vi "AFXP Main.vi"() -> ()   [LabVIEW 2015]
doc: "Simple File Manager for the Adafruid Audio FX Sound Board\nhttps://learn.adafruit.com/adafruit-audio-fx-sound-board/overview"
uses:
  controls/AFXP State.ctl
  controls/AFXP Data.ctl
  controls/AFCP Setup.ctl
  <vilib>/Utility/error.llb/DialogType.ctl
  <userlib>/_OpenG.lib/file/file.llb/File Exists - Scalar__ogtk.vi
panel:
  in  "Clear Button":bool
  in  "Button Ctrl":T1={"Trigger Type:"=enum."Disabled", "Sound Files"=[]}
  in  "Folder Drop":path
  in  "Prev Button":bool
  in  "Next Button":bool
  in  "Button Selection":T2(ring)
  in  "Make Button":bool
  in  "Destination":path
  # "AUDIO FILE LIST"
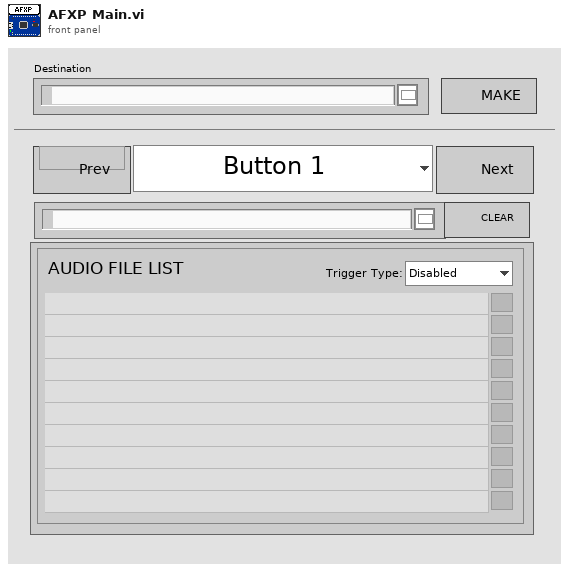
[diagram p1: front panel]
types:
  T1 = cluster{"Trigger Type:":enum16{"Basic", "Hold-Loop", "Latch-Loop", "Next", "Random", "Disabled"}, "Sound Files":path[]}
  T2 = enum8{"Button 1", "Button 2", "Button 3", "Button 4", "Button 5", "Button 6", "Button 7", "Button 8", "Button 9", "Button 10", "Button 11", "Button 12"}
  T3 = typedef "AFXP Data.ctl" = cluster{"changes_saved?":bool, "button_setup":T4[], "Destination":path}
  T4 = typedef "AFCP Setup.ctl" = cluster{"trigger":enum16{"Basic", "Hold-Loop", "Latch-Loop", "Next", "Random", "Disabled"}, "files":path[]}
  T5 = typedef "AFXP State.ctl" = enum16{"Initialize", "Wait for Event", "Make", "Load", "Save", "Folder Drop", "Prev", "Next", "Button Ctrl", "Destination", "Selection", "Exit"}
  T6 = cluster{"Trigger Type":enum16{"Basic", "Hold-Loop", "Latch-Loop", "Next", "Random", "Disabled"}, "Sound Files":path[]}
  T7 = typedef "DialogType.ctl" = u16
  T8 = cluster{"Trigger Type":enum16{"Basic", "Hold-Loop", "Latch-Loop", "Next", "Random", "Disabled"}, "Sound Files":path[]}[]
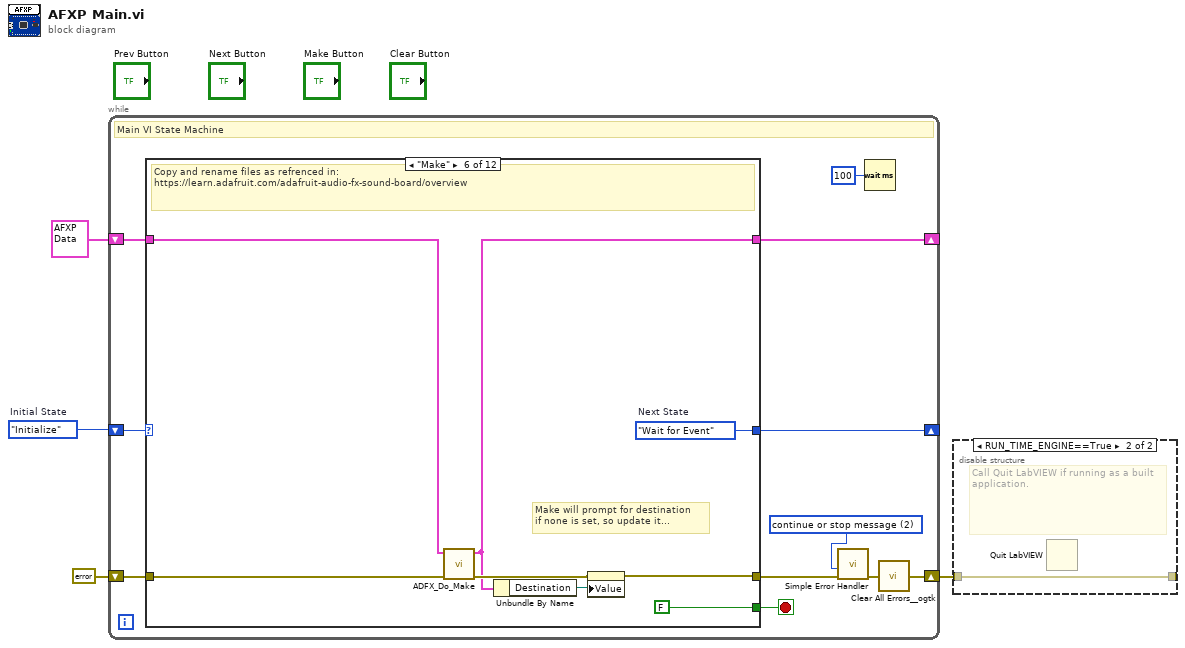
[diagram p0: block diagram]
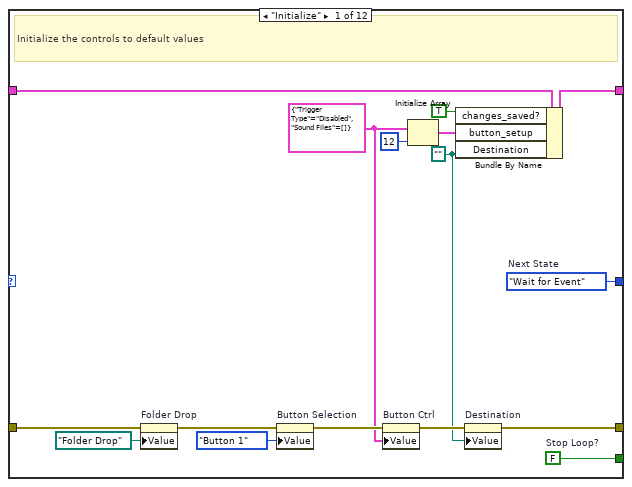
[diagram p2: hidden frame]
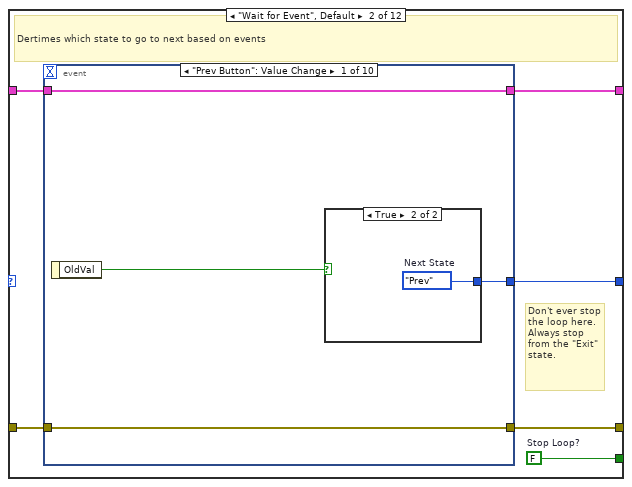
[diagram p3: hidden frame]
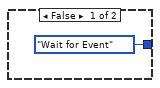
[diagram p4: hidden frame]
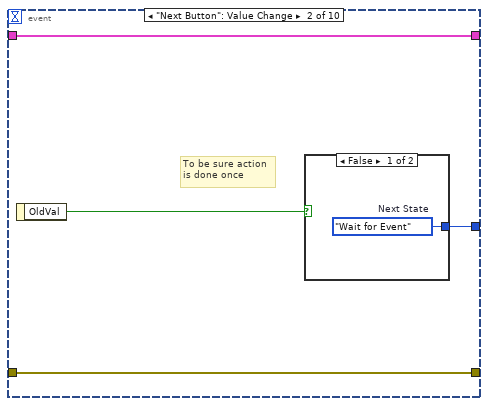
[diagram p5: hidden frame]
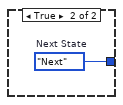
[diagram p6: hidden frame]
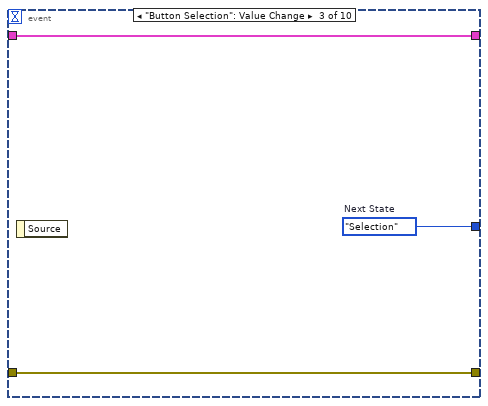
[diagram p7: hidden frame]
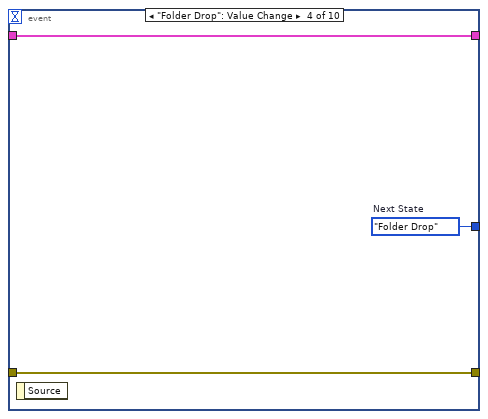
[diagram p8: hidden frame]
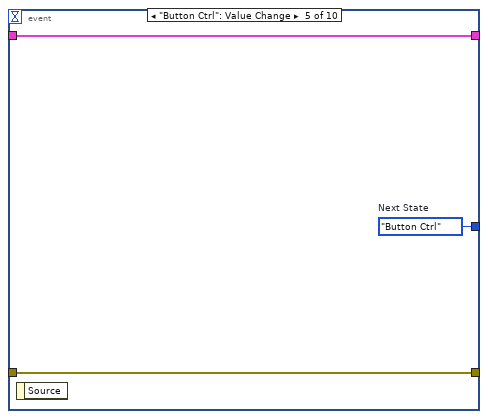
[diagram p9: hidden frame]
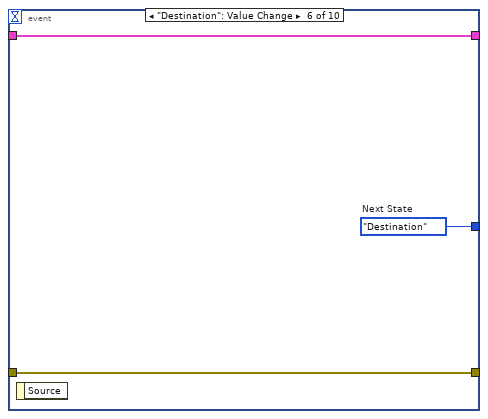
[diagram p10: hidden frame]
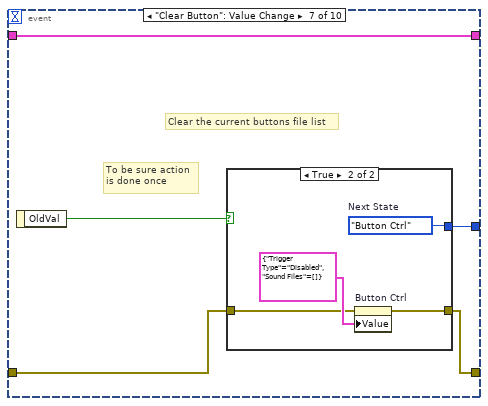
[diagram p11: hidden frame]
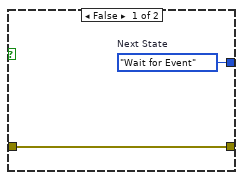
[diagram p12: hidden frame]
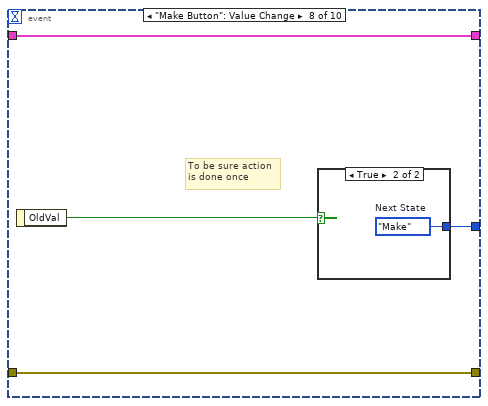
[diagram p13: hidden frame]
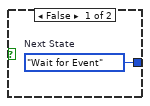
[diagram p14: hidden frame]
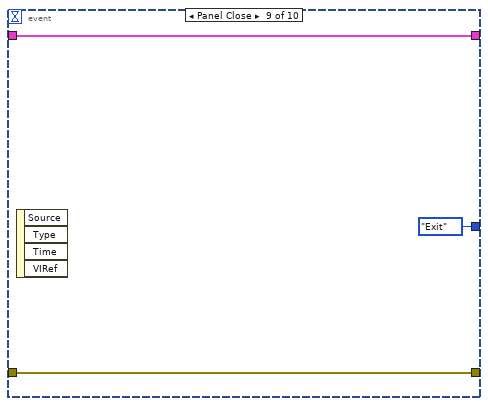
[diagram p15: hidden frame]
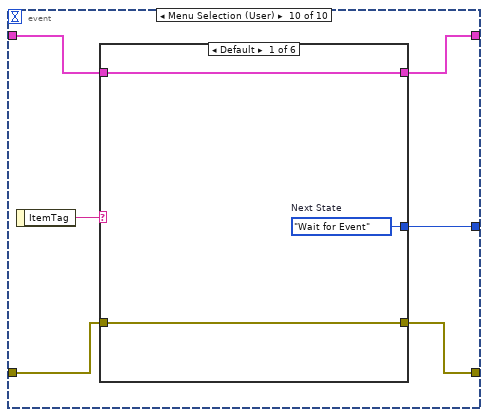
[diagram p16: hidden frame]
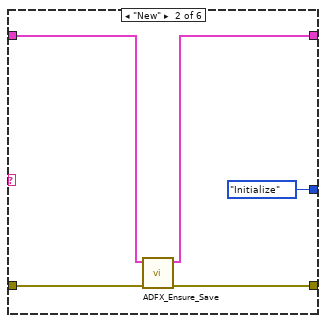
[diagram p17: hidden frame]
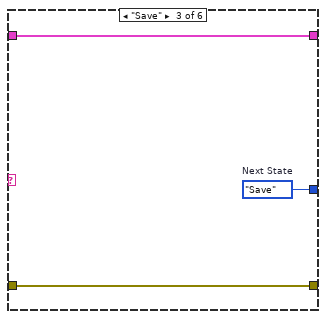
[diagram p18: hidden frame]
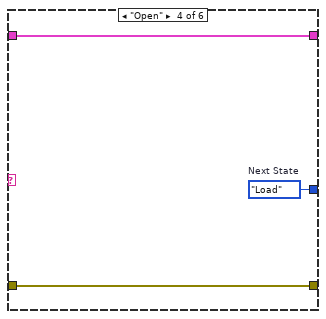
[diagram p19: hidden frame]
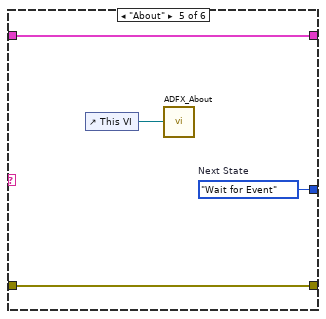
[diagram p20: hidden frame]
diagram:
  w4 = AFXP_State."Initialize"  # Initial State
  n1 = while {
    shift-right: [w14] -> _
    shift-left: w4 -> [w15]
    shift-right: [w12] -> _
    shift-left: T3 {"changes_saved?"=TRUE, "button_setup"=[{"trigger"=enum."Basic", "files"=[]}, {"trigger"=enum."Basic", "files"=[]}, {"trigger"=enum."Basic", "files"=[]}, {"trigger"=enum."Basic", "files"=[]}, {"trigger"=enum."Basic", "files"=[]}, {"trigger"=enum."Basic", "files"=[]}, {"trigger"=enum."Basic", "files"=[]}, {"trigger"=enum."Basic", "files"=[]}, {"trigger"=enum."Basic", "files"=[]}, {"trigger"=enum."Basic", "files"=[]}, {"trigger"=enum."Basic", "files"=[]}, {"trigger"=enum."Basic", "files"=[]}, {"trigger"=enum."Basic", "files"=[]}], "Destination"=path ""} ("Data") -> [w13]
    shift-right: [w5] -> w1
    shift-left: errorcluster {"status"=FALSE, "code"=0, "source"=""} ("error constant") -> [w11]
    stop <- w6 stop-if-true
    w7 = T7 2 items=["no dialog", "OK message", "continue or stop message", "OK message + warnings", "continue/stop + warnings"] ("type of dialog (OK msg:1)")
    # "Main VI State Machine"
    n2 = case shown="\"Make\"" w15 {
      tunnel: [w31 w37 w114 w115 w133 w142 w160 w170 w171 w179 w187 w206] -> w14
      tunnel: [w30 w36 FALSE ("Stop Loop?") FALSE ("Stop Loop?") FALSE ("Stop Loop?") FALSE ("Stop Loop?") FALSE ("Stop Loop?") w169 FALSE ("Stop Loop?") FALSE ("Stop Loop?") FALSE ("Stop Loop?") FALSE ("Stop Loop?")] -> w6
      tunnel: w13 -> [w24 w35 w110 w120 w134 w139 w158 w166 w178 w186 w198 w205]
      tunnel: [w23 w34 w109 w116 w132 w136 w158 w165 w178 w186 w197 w205] -> w12
      tunnel: w11 -> [w29 w33 w111 w122 w126 w140 w157 w168 w176 w182 w194 w202]
      tunnel: [w17 w32 w112 w118 w125 w137 w151 w167 w172 w180 w191 w204] -> w9
      frame "Initialize" {
        w16 = path ""
        w20 = T6 {"Trigger Type"=enum."Disabled", "Sound Files"=[]} ("Button Ctrl")
        w30 = FALSE  # Stop Loop?
        w31 = AFXP_State."Wait for Event"  # Next State
        # "Initialize the controls to default values"
        n3 = property on="Folder Drop" class="Path"(error in=w29, "Value"=path "Folder Drop" ("Destination")) -> (error out=w26:errorcluster)  [unwired: 1 in, 1 out]
        n4 = property on="Button Selection" class="Enum (strict)"(error in=w26, "Value"=T2."Button 1" ("Button Selection")) -> (error out=w25:errorcluster)  [unwired: 1 in, 1 out]
        n5 = property on="Button Ctrl" class="Clust (strict)"(error in=w25, "Value"=w20) -> (error out=w18:errorcluster)  [unwired: 1 in, 1 out]
        n6 = Initialize Array(w20, 12 ("dimension size")) -> (w21:T8)
        n7 = Bundle By Name(cluster=w24, "changes_saved?"=TRUE, "button_setup"=w21, "Destination"=w16) -> (w23:T3)
        n8 = property on="Destination" class="Path"(error in=w18, "Value"=w16) -> (error out=w17:errorcluster)  [unwired: 1 in, 1 out]
      }
      frame "Wait for Event", Default {
        w36 = FALSE  # Stop Loop?
        # "Don't ever stop the loop here. Always stop from the \"Exit\" state."
        # "Dertimes which state to go to next based on events"
        n9 = event shown="[0] \"Prev Button\": Value Change" {
          selector: _ -> [_ _ _ _ _ _ _ _ _ _]
          dyn-events: _ -> [_ _ _ _ _ _ _ _ _ _]
          timeout: _ -> [_ _ _ _ _ _ _ _ _ _]
          tunnel: [w41 w45 w50 w53 w56 w59 w65 w74 AFXP_State."Exit" ("Next State") w86] -> w37
          tunnel: w35 -> [w40 w47 w52 w55 w58 w61 w66 w76 w81 w83]
          tunnel: [w40 w47 w52 w55 w58 w61 w66 w76 w81 w82] -> w34
          tunnel: w33 -> [w39 w46 w51 w54 w57 w60 w63 w75 w80 w85]
          tunnel: [w39 w46 w51 w54 w57 w60 w62 w75 w80 w84] -> w32
          event "Prev Button": Value Change {
            n10 = event-data() -> ("OldVal"=w38:bool)  [unwired: 1 in]
            n11 = case shown="True" w38 {
              tunnel: [AFXP_State."Wait for Event" ("Next State") w43] -> w41
              frame False {
              }
              frame True {
                w43 = AFXP_State."Prev"  # Next State
              }
            }
          }
          event "Next Button": Value Change {
            # "To be sure action\nis done once"
            n12 = event-data() -> ("OldVal"=w44:bool)  [unwired: 1 in]
            n13 = case shown="False" w44 {
              tunnel: [w48 w49] -> w45
              frame False {
                w48 = AFXP_State."Wait for Event"  # Next State
              }
              frame True {
                w49 = AFXP_State."Next"  # Next State
              }
            }
          }
          event "Button Selection": Value Change {
            w50 = AFXP_State."Selection"  # Next State
            n14 = event-data() -> ()  [unwired: 1 in, 1 out]
          }
          event "Folder Drop": Value Change {
            w53 = AFXP_State."Folder Drop"  # Next State
            n15 = event-data() -> ()  [unwired: 1 in, 1 out]
          }
          event "Button Ctrl": Value Change {
            w56 = AFXP_State."Button Ctrl"  # Next State
            n16 = event-data() -> ()  [unwired: 1 in, 1 out]
          }
          event "Destination": Value Change {
            w59 = AFXP_State."Destination"  # Next State
            n17 = event-data() -> ()  [unwired: 1 in, 1 out]
          }
          event "Clear Button": Value Change {
            # "To be sure action\nis done once"
            # "Clear the current buttons file list"
            n18 = event-data() -> ("OldVal"=w64:bool)  [unwired: 1 in]
            n19 = case shown="True" w64 {
              tunnel: [w68 w72] -> w65
              tunnel: w63 -> [w67 w70]
              tunnel: [w67 w69] -> w62
              frame False {
                w68 = AFXP_State."Wait for Event"  # Next State
              }
              frame True {
                w72 = AFXP_State."Button Ctrl"  # Next State
                n20 = property on="Button Ctrl" class="Clust (strict)"(error in=w70, "Value"=T6 {"Trigger Type"=enum."Disabled", "Sound Files"=[]} ("Button Ctrl")) -> (error out=w69:errorcluster)  [unwired: 1 in, 1 out]
              }
            }
          }
          event "Make Button": Value Change {
            # "To be sure action\nis done once"
            n21 = event-data() -> ("OldVal"=w73:bool)  [unwired: 1 in]
            n22 = case shown="True" w73 {
              tunnel: [w77 w78] -> w74
              frame False {
                w77 = AFXP_State."Wait for Event"  # Next State
              }
              frame True {
                w78 = AFXP_State."Make"  # Next State
              }
            }
          }
          event Panel Close {
            n23 = event-data() -> ()  [unwired: 1 in, 4 out]
          }
          event Menu Selection (User) {
            n24 = event-data() -> ("ItemTag"=w87:string)  [unwired: 1 in]
            n25 = case shown="Default" w87 {
              tunnel: [w90 AFXP_State."Initialize" ("Next State") w98 w101 w105 AFXP_State."Exit" ("Next State")] -> w86
              tunnel: w85 -> [w89 w94 w97 w100 w103 w107]
              tunnel: [w89 w93 w97 w100 w103 w107] -> w84
              tunnel: w83 -> [w88 w92 w96 w99 w104 w106]
              tunnel: [w88 w91 w96 w99 w104 w106] -> w82
              frame Default {
                w90 = AFXP_State."Wait for Event"  # Next State
              }
              frame "New" {
                n26 = call "ADFX_Ensure_Save.vi"("error in (no error)"=w94, "Data in"=w92) -> ("error out"=w93:errorcluster, "Data out"=w91:T3)  [unwired: 8 in]
              }
              frame "Save" {
                w98 = AFXP_State."Save"  # Next State
              }
              frame "Open" {
                w101 = AFXP_State."Load"  # Next State
              }
              frame "About" {
                w105 = AFXP_State."Wait for Event"  # Next State
                n27 = control-ref of="This VI"() -> (w102:refnum<vi>)
                n28 = call "ADFX_About.vi"("reference"=w102) -> ()
              }
              frame "Exit" {
              }
            }
          }
        }
      }
      frame "Save" {
        w114 = AFXP_State."Wait for Event"  # Next State
        # "Save the setup data"
        n29 = call "ADFX_Do_Save.vi"("error in (no error)"=w111, "Data in"=w110) -> ("error out"=w112:errorcluster, "Data out"=w109:T3)  [unwired: 8 in]
      }
      frame "Load" {
        w115 = AFXP_State."Selection"  # Next State
        # "Button selection will update\ncontrols"
        # "Update destination here since it\nisn't necessary to do it every time we\nchange button selection."
        # "Load the setup data"
        n30 = call "ADFX_Ensure_Save.vi"("error in (no error)"=w122, "Data in"=w120) -> ("error out"=w123:errorcluster, "Data out"=w121:T3)  [unwired: 8 in]
        n31 = call "ADFX_Do_Load.vi"("error in (no error)"=w123, "Data in"=w121) -> ("error out"=w119:errorcluster, "Data out"=w116:T3)  [unwired: 8 in]
        n32 = Unbundle By Name(w116) -> ("Destination"=w117:path)
        n33 = property on="Destination" class="Path"(error in=w119, "Value"=w117) -> (error out=w118:errorcluster)  [unwired: 1 in, 1 out]
      }
      frame "Destination" {
        w133 = AFXP_State."Wait for Event"  # Next State
        # "Set destination unless empty, then make sure it knows it's empty."
        n34 = Empty String/Path?(string/path="Destination") -> (empty?=w130:bool)
        n35 = Select(t=path "", s=w130, f="Destination") -> (s? t:f=w127:path)
        n36 = Bundle By Name(cluster=w134, "Destination"=w127) -> (w132:T3)
        n37 = property on="Destination" class="Path"(error in=w126, "Value"=w127) -> (error out=w125:errorcluster)  [unwired: 1 in, 1 out]
      }
      frame "Make" {
        w142 = AFXP_State."Wait for Event"  # Next State
        # "Make will prompt for destination\nif none is set, so update it..."
        # "Copy and rename files as refrenced in:\nhttps://learn.adafruit.com/adafruit-audio-fx-sound-board/overview"
        n38 = call "ADFX_Do_Make.vi"("error in (no error)"=w140, "Data in"=w139) -> ("error out"=w138:errorcluster, "Data out"=w136:T3)  [unwired: 8 in]
        n39 = Unbundle By Name(w136) -> ("Destination"=w135:path)
        n40 = property on="Destination" class="Path"(error in=w138, "Value"=w135) -> (error out=w137:errorcluster)  [unwired: 1 in, 1 out]
      }
      frame "Folder Drop" {
        w160 = AFXP_State."Button Ctrl"  # Next State
        # "Go to button control as it\nchecks files in list"
        # "get files directory if file"
        # "Add files in directory to current button selected."
        n41 = call-poly <userlib>:"File Exists__ogtk.vi"("file path"="Folder Drop") -> ("is directory"=w146:bool)  [unwired: 6 in, 1 out]
        n42 = Strip Path(path="Folder Drop") -> (stripped path=w144:path)  [unwired: 1 out]
        n43 = Select(t="Folder Drop", s=w146, f=w144) -> (s? t:f=w143:path)
        n44 = call <userlib>:"List Directory__ogtk.vi"("error in (no error)"=w157, "pattern"="*.ogg;*.wav", "directory path"=w143) -> ("error out"=w161:errorcluster, "file names"=w149:string[], "dup directory path"=w156:path)  [unwired: 1 in, 1 out]
        n45 = for {
          tunnel: w156 -> [w164]
          tunnel: w149 -> [w163] mode=indexing
          tunnel: [w162] -> w154 mode=indexing
          n46 = Build Path(base path=w164, name or relative path=w163) -> (appended path=w162:path)
        }
        n47 = property on="Sound Files" class="Arr (strict)"(error in=w161) -> (error out=w153:errorcluster, "Value"=w155:path[])  [unwired: 1 in, 1 out]
        n48 = Insert Into Array(array=w155, new element=w154) -> (w148:path[])  [unwired: 1 in]
        n49 = property on="Sound Files" class="Arr (strict)"(error in=w153, "Value"=w148) -> (error out=w150:errorcluster)  [unwired: 1 in, 1 out]
        n50 = property on="Folder Drop" class="Path"(error in=w150, "Value"=path "Folder Drop" ("Destination")) -> (error out=w151:errorcluster)  [unwired: 1 in, 1 out]
      }
      frame "Exit" {
        w169 = TRUE  # Stop Loop?
        w170 = AFXP_State."Exit"  # (Value Not Used)
        # "Exit - Exit the application."
        n51 = call "ADFX_Ensure_Save.vi"("error in (no error)"=w168, "Data in"=w166) -> ("error out"=w167:errorcluster, "Data out"=w165:T3)  [unwired: 8 in]
      }
      frame "Prev" {
        w171 = AFXP_State."Selection"  # Next State
        # "go to previous button selection"
        n52 = property on="Button Selection" class="Enum (strict)"(error in=w176) -> (error out=w177:errorcluster, "Value"=w175:T2)  [unwired: 1 in, 1 out]
        n53 = Decrement(x=w175) -> (x-1=w174:T2)
        n54 = property on="Button Selection" class="Enum (strict)"(error in=w177, "Value"=w174) -> (error out=w172:errorcluster)  [unwired: 1 in, 1 out]
      }
      frame "Next" {
        w179 = AFXP_State."Selection"  # Next State
        # "go to the next button selection"
        n55 = property on="Button Selection" class="Enum (strict)"(error in=w182) -> (error out=w185:errorcluster, "Value"=w184:T2)  [unwired: 1 in, 1 out]
        n56 = Increment(x=w184) -> (x+1=w183:T2)
        n57 = property on="Button Selection" class="Enum (strict)"(error in=w185, "Value"=w183) -> (error out=w180:errorcluster)  [unwired: 1 in, 1 out]
      }
      frame "Button Ctrl" {
        w187 = AFXP_State."Selection"  # Next State
        # "Handle Button Control Changes"
        n58 = Unbundle By Name(w198) -> ("button_setup"=w196:T4[])
        n59 = property on="Button Selection" class="Enum (strict)"(error in=w194) -> (error out=w193:errorcluster, "Value"=w190:T2)  [unwired: 1 in, 1 out]
        n60 = call "Button_Ctrl_Check.vi"("error in (no error)"=w193, "Button Ctrl in"="Button Ctrl") -> ("error out"=w191:errorcluster, "Button Ctrl out"=w189:T6)  [unwired: 8 in]
        n61 = Replace Array Subset(array=w196, new element=w189, index=w190) -> (w195:T4[])
        n62 = Bundle By Name(cluster=w198, "changes_saved?"=FALSE, "button_setup"=w195) -> (w197:T3)
      }
      frame "Selection" {
        w206 = AFXP_State."Wait for Event"  # Next State
        n63 = Unbundle By Name(w205) -> ("button_setup"=w203:T4[])
        n64 = Index Array(array=w203, index="Button Selection") -> (element=w200:T4)
        n65 = property on="Button Ctrl" class="Clust (strict)"(error in=w202, "Value"=w200) -> (error out=w204:errorcluster)  [unwired: 1 in, 1 out]
      }
    }
    n66 = call <vilib>:"Simple Error Handler.vi"("type of dialog (OK msg:1)"=w7, "error in (no error)"=w9) -> ("error out"=w8:errorcluster)  [unwired: 3 in, 4 out]
    n67 = Wait (ms)(milliseconds to wait=u32 100) -> ()  [unwired: 1 out]
    n68 = call <userlib>:"Clear All Errors__ogtk.vi"("Error In"=w8) -> ("Error Out"=w5:errorcluster)  [unwired: 3 in]
  }
  n69 = disable-structure shown="RUN_TIME_ENGINE==True" {
    disable-tunnel: [w208 w209] -> _
    disable-tunnel: w1 -> [w208 w209]
    frame condition #0 (active) {
    }
    frame condition #1 {
      # "Call Quit LabVIEW if running as a built application."
      n70 = Quit LabVIEW() -> ()  [unwired: 1 in]
    }
  }
